vi "example test.vi"() -> ()   [LabVIEW 2013, in "Profibus Module tests.lvlib"]
uses:
  Profibus Module tests.lvlib
  configuration/Profibus Module configuration.lvclass
  execution/Profibus Module runtime.lvclass
  <vilib>/NI/Tag Bus/dictionary/data dictionary.lvclass
  <vilib>/NI/Tag Bus/table/data table.lvlib
  channel/Profibus channel.lvclass
  <vilib>/NI/Tag Bus/tag/Data Type.ctl
  <vilib>/NI/Tag Bus/tag/tag descriptor.lvclass
  <vilib>/NI/Tag Bus Module Framework/channel/channel classification.ctl
  <vilib>/NI/Tag Bus Module Framework/channel/TBM channel.lvclass
  <vilib>/NI/Tag Bus/dictionary/lookup polymorphs/locate Boolean.vi
  <vilib>/NI/Tag Bus/table/data polymorphs/write one/write Boolean.vi
  <vilib>/NI/Tag Bus/table/data polymorphs/read one/read Boolean.vi
panel:
  in  "DO bit":i32
  in  "DO byte":i32
  in  "DI bit":i32
  in  "DI byte":i32
  in  "stop":bool
  in  "DO":bool
  out "DI":bool
  out "final error":errorcluster
  out "output error":errorcluster
  out "input error":errorcluster
  out "output lookup error":errorcluster
  out "input lookup error":errorcluster
  out "init error":errorcluster
  out "correct execution settings":bool
  out "serialization problem":errorcluster
  out "invalid configuration":errorcluster
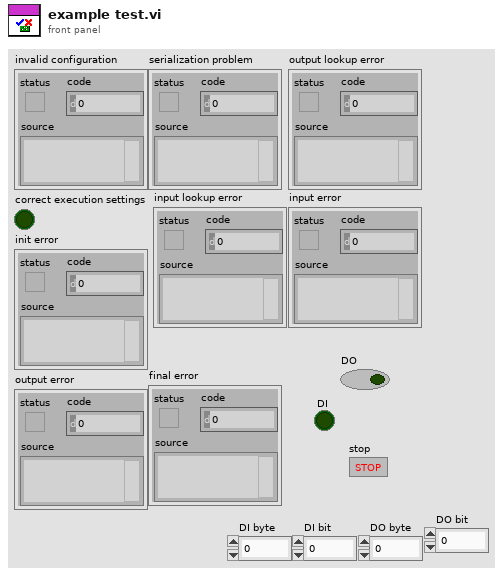
[diagram p1: front panel]
types:
  T1 = typedef "TBM channel.lvclass/channel classification.ctl" = enum16{"input data", "output data", "processing parameter", "processing result"}
  T2 = typedef "tag bus.lvlib/tag descriptor.lvclass/Data Type.ctl" = enum16{"Double", "Single", "I64", "I32", "I16", "I8", "U64", "U32", "U16", "U8", "Boolean", "String", "Array of Double", "Array of Single", "Array of I64", "Array of I32", "Array of I16", "Array of I8", "Array of U64", "Array of U32", "Array of U16", "Array of U8", "Array of Boolean", "Array of String"}
  T3 = typedef "TBM channel.lvclass/data tables.ctl" = cluster{"input data":T4, "processing parameter":T4, "processing result":T4, "output data":T4}
  T4 = typedef "tag bus.lvlib/dictionary table pair.ctl" = cluster{"data dictionary":refnum<class "data dictionary.lvclass">, "data table":T5}
  T5 = typedef "tag bus.lvlib/data table.lvlib/data table.ctl" = cluster{"Double":dbl[], "Single":sgl[], "I64":i64[], "I32":i32[], "I16":i16[], "I8":i8[], "U64":u64[], "U32":u32[], "U16":u16[], "U8":u8[], "Boolean":bool[], "String":string[], "Array of Double":cluster{"DBL Array":dbl[]}[], "Array of Single":cluster{"SGL Array":sgl[]}[], "Array of I64":cluster{"I64 Array":i64[]}[], "Array of I32":cluster{"I32 Array":i32[]}[], "Array of I16":cluster{"I16 Array":i16[]}[], "Array of I8":cluster{"I8 Array":i8[]}[], "Array of U64":cluster{"U64 Array":u64[]}[], "Array of U32":cluster{"U32 Array":u32[]}[], "Array of U16":cluster{"U16 Array":u16[]}[], "Array of U8":cluster{"U8 Array":u8[]}[], "Array of Boolean":cluster{"Boolean Array":bool[]}[], "Array of String":cluster{"String Array":string[]}[]}
  T6 = typedef "TBM module execution interface.lvclass/execution settings.ctl" = cluster{"reads inputs":bool, "processes data":bool, "writes outputs":bool}
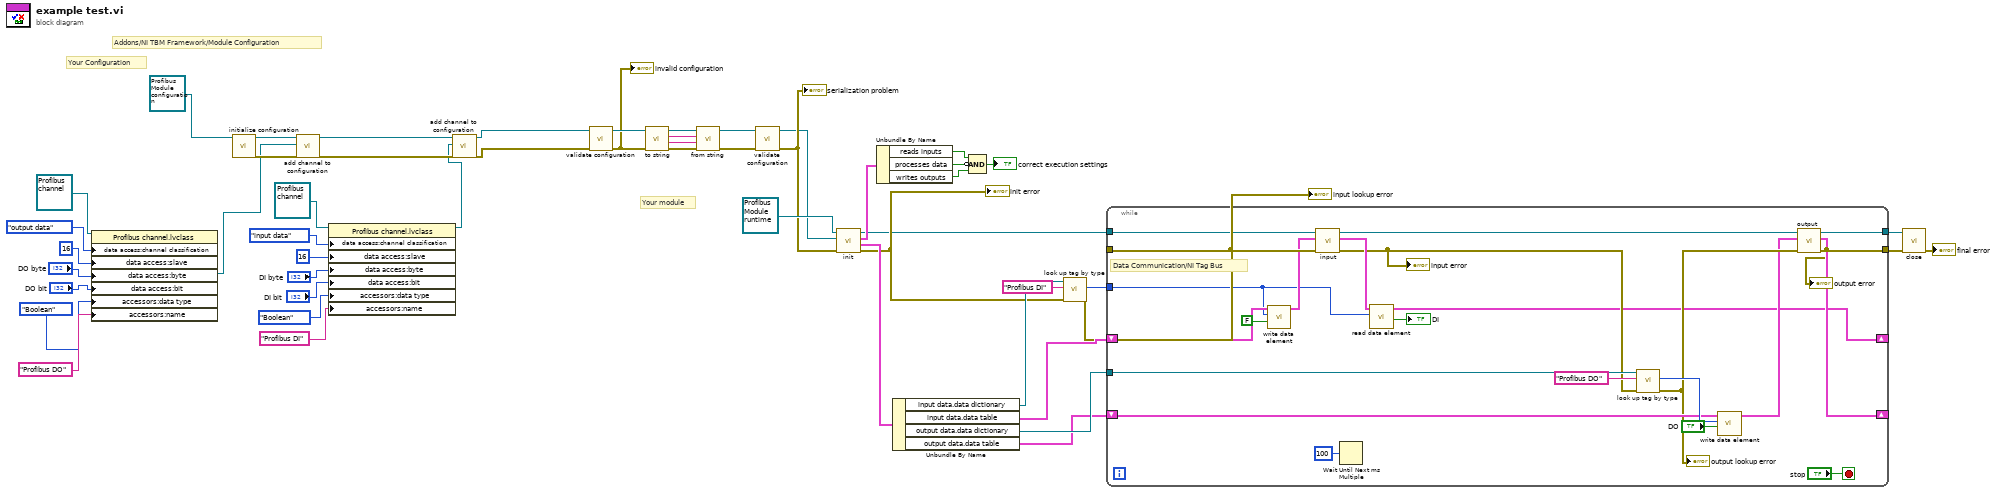
[diagram p0: block diagram]
diagram:
  # "Your Configuration"
  # "Addons/NI TBM Framework/Module Configuration"
  # "Your module"
  n1 = property class="Profibus channel.lvclass"(reference=refnum<class "Profibus channel.lvclass"> refnum ("Profibus channel.lvclass"), "data access:channel classification"=channel_classification."output data" ("channel classification"), "data access:slave"=i8 16 ("slave"), "data access:byte"="DO byte", "data access:bit"="DO bit", "accessors:data type"=Data_Type."Boolean" ("data type"), "accessors:name"="Profibus DO" ("name")) -> (reference out=w1:refnum<class "Profibus channel.lvclass">)  [unwired: 1 in, 1 out]
  n2 = call-dynamic "initialize configuration.vi"("configuration in"=refnum<class "Profibus Module configuration.lvclass"> refnum ("tag bus configurable plugin module configuration")) -> ("error out"=w17:errorcluster, "configuration out"=w18:refnum<class "Profibus Module configuration.lvclass">)  [unwired: 8 in, 1 out]
  n3 = call "add channel to configuration.vi"("error in"=w17, "TBM channel in"=w1, "Profibus Module configuration in"=w18) -> ("error out"=w19:errorcluster, "Profibus Module configuration out"=w20:refnum<class "Profibus Module configuration.lvclass">)  [unwired: 7 in]
  n4 = property class="Profibus channel.lvclass"(reference=refnum<class "Profibus channel.lvclass"> refnum ("Profibus channel.lvclass"), "data access:channel classification"=channel_classification."input data" ("channel classification"), "data access:slave"=i8 16 ("slave"), "data access:byte"="DI byte", "data access:bit"="DI bit", "accessors:data type"=Data_Type."Boolean" ("data type"), "accessors:name"="Profibus DI" ("name")) -> (reference out=w2:refnum<class "Profibus channel.lvclass">)  [unwired: 1 in, 1 out]
  n5 = call "add channel to configuration.vi"("error in"=w19, "TBM channel in"=w2, "Profibus Module configuration in"=w20) -> ("error out"=w22:errorcluster, "Profibus Module configuration out"=w23:refnum<class "Profibus Module configuration.lvclass">)  [unwired: 7 in]
  n6 = call-dynamic "validate configuration.vi"("error in"=w22, "Profibus Module configuration in"=w23) -> ("error out"=w51:errorcluster, "Profibus Module configuration out"=w52:refnum<class "Profibus Module configuration.lvclass">)  [unwired: 8 in]
  "invalid configuration" <- w51
  n7 = call-dynamic "to string.vi"("error in"=w51, "Profibus Module configuration in"=w52) -> ("error out"=w47:errorcluster, "data"=w48:string, "version"=w49:string, "Profibus Module configuration out"=w50:refnum<class "Profibus Module configuration.lvclass">)  [unwired: 6 in]
  n8 = call-dynamic "from string.vi"("error in"=w47, "data"=w48, "version"=w49, "Profibus Module configuration in"=w50) -> ("error out"=w45:errorcluster, "Profibus Module configuration out"=w46:refnum<class "Profibus Module configuration.lvclass">)  [unwired: 6 in]
  n9 = call-dynamic "validate configuration.vi"("error in"=w45, "Profibus Module configuration in"=w46) -> ("error out"=w43:errorcluster, "Profibus Module configuration out"=w42:refnum<class "Profibus Module configuration.lvclass">)  [unwired: 8 in]
  "serialization problem" <- w43
  n10 = call-dynamic "init.vi"("error in"=w43, "TBM module configuration in"=w42, "Profibus Module runtime in"=refnum<class "Profibus Module runtime.lvclass"> refnum ("tag bus configurable plugin module")) -> ("error out"=w34:errorcluster, "data allocations"=w36:T3, "execution settings"=w41:T6, "Profibus Module runtime out"=w31:refnum<class "Profibus Module runtime.lvclass">)  [unwired: 5 in]
  "init error" <- w34
  n11 = Unbundle By Name(w41) -> ("reads inputs"=w38:bool, "processes data"=w40:bool, "writes outputs"=w39:bool)
  n12 = Unbundle By Name(w36) -> ("input data.data dictionary"=w35:refnum<class "data dictionary.lvclass">, "input data.data table"=w32:T5, "output data.data dictionary"=w28:refnum<class "data dictionary.lvclass">, "output data.data table"=w27:T5)
  n13 = Compound Arithmetic op=AND(w38, invert w40, w39) -> (→"correct execution settings":bool)
  n14 = call-poly <vilib>:"look up tag by type.vi"("error in"=w34, "name"="Profibus DI" ("channel name"), "data dictionary in"=w35) -> ("error out"=w30:errorcluster, "index"=w29:i32)  [unwired: 6 in, 1 out]
  "input lookup error" <- w30
  n15 = while {
    tunnel: w31 -> [w74]
    tunnel: w30 -> [w73]
    tunnel: w29 -> [w70]
    tunnel: w28 -> [w69]
    tunnel: [w61] -> w26
    tunnel: [w53] -> w25
    shift-right: [w57] -> _
    shift-left: w27 -> [w66]
    shift-right: [w56] -> _
    shift-left: w32 -> [w75]
    stop <- "stop" stop-if-true
    # "Data Communication/NI Tag Bus"
    n16 = call-poly <vilib>:"write data element.vi"("value"=FALSE, "index"=w70, "data table in"=w75) -> ("data table out"=w72:T5)  [unwired: 8 in]
    n17 = call-dynamic "input.vi"("error in"=w73, "data table in"=w72, "Profibus Module runtime in"=w74) -> ("error out"=w65:errorcluster, "data table out"=w71:T5, "Profibus Module runtime out"=w63:refnum<class "Profibus Module runtime.lvclass">)  [unwired: 6 in]
    "input error" <- w65
    n18 = Wait Until Next ms Multiple(millisecond multiple=u32 100) -> ()  [unwired: 1 out]
    n19 = call-poly <vilib>:"read data element.vi"("index"=w70, "data table in"=w71) -> ("value"=→"DI":bool, "data table out"=w56:T5)  [unwired: 8 in]
    n20 = call-poly <vilib>:"look up tag by type.vi"("error in"=w65, "name"="Profibus DO" ("channel name"), "data dictionary in"=w69) -> ("error out"=w64:errorcluster, "index"=w67:i32)  [unwired: 6 in, 1 out]
    "output lookup error" <- w64
    n21 = call-poly <vilib>:"write data element.vi"("value"="DO", "index"=w67, "data table in"=w66) -> ("data table out"=w62:T5)  [unwired: 8 in]
    n22 = call-dynamic "output.vi"("error in"=w64, "data table in"=w62, "Profibus Module runtime in"=w63) -> ("error out"=w53:errorcluster, "data table out"=w57:T5, "Profibus Module runtime out"=w61:refnum<class "Profibus Module runtime.lvclass">)  [unwired: 6 in]
    "output error" <- w53
  }
  n23 = call-dynamic "close.vi"("error in"=w25, "Profibus Module runtime in"=w26) -> ("error out"=→"final error":errorcluster)  [unwired: 9 in]
